vi "Normalize Scheme Port.vi"(4 "URI in":refnum<class "URI.lvclass">) -> (7 "URI out":refnum<class "URI.lvclass">)   [LabVIEW 2020, in "URI.lvlib" / "URI.lvclass"]
uses:
  URI.lvclass
  URI.lvclass/URI.ctl
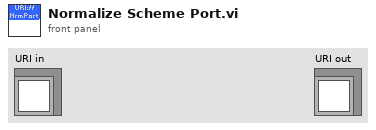
[diagram p1: front panel]
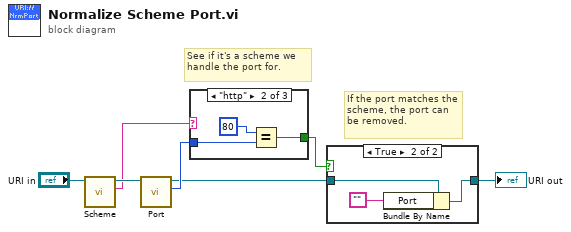
[diagram p0: block diagram]
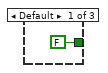
[diagram p3: hidden frame]
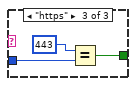
[diagram p4: hidden frame]
diagram:
  # "If the port matches the scheme, the port can be removed."
  # "See if it's a scheme we handle the port for."
  n1 = call "Scheme.vi"("URI in"="URI in") -> ("Scheme"=w6:string, "URI out"=w7:refnum<class "URI.lvclass">)  [unwired: 9 in]
  n2 = call "Port.vi"("URI in"=w7) -> ("Port"=w5:u16, "URI out"=w4:refnum<class "URI.lvclass">)  [unwired: 8 in, 1 out]
  n3 = case shown="\"http\"" w6 {
    tunnel: w5 -> [_ w11 w14]
    tunnel: [FALSE w9 w12] -> w3
    frame Default {
    }
    frame "http" {
      n4 = Equal?(x=u16 80 ("y"), y=w11) -> (x = y?=w9:bool)
    }
    frame "https" {
      n5 = Equal?(x=u16 443 ("y"), y=w14) -> (x = y?=w12:bool)
    }
  }
  n6 = case shown="True" w3 {
    tunnel: w4 -> [w15 w18]
    tunnel: [w15 w16] -> w1
    frame False {
    }
    frame True {
      n7 = Bundle By Name(cluster=w18, "Port"="") -> (w16:refnum<class "URI.lvclass">)
    }
  }
  "URI out" <- w1
